vi "Keithley 2002 ACI Config.vi"(0 "GPIB address":string="16", 1 "integration time (0:auto)":u16(ring) items=["automatic", "automatic once", "set to minimum", "set to maximum", "set aperature value", "set NPLC value"], 2 "integ. value":dbl=0.01667 format="%^.2e", 3 "range (auto:0)":u16(ring) items=["autorange", "autorange once", "set min range", "set max range", "set range value"], 4 "range value (amps)":dbl=2.0 min=0.0002 max=2.0 format="%^.2e", 5 "error in":T1, 6 "coupling":bool=TRUE, 7 "resolution (4.5 digits:3)":u16(ring)=3 items=["auto resolution", "auto resolution once", "3.5 digits", "4.5 digits", "5.5 digits", "6.5 digits", "7.5 digits", "8.5 digits"], 8 "reference (off:0)":u16(ring) items=["off", "set reference value"], 9 "digital filter (off:0)":u16(ring) items=["off", "auto filter", "auto filter once", "moving filter", "repeating filter"], 10 "reference value (amps)":dbl min=-2.1 max=2.1 format="%^.2e", 11 "dig. filter count":dbl=10.0 min=1.0 max=100.0 step=1.0 format="%^.2e", 14 "advanced filter (off:0)":u16(ring) items=["off", "enabled"], 15 "noise tolerance (%)":dbl=5.0 min=0.0 max=100.0 step=1.0 format="%^.2e", 16 "detector (rms:0)":u16(ring) items=["RMS", "average"]) -> (19 "error out":T1)   [LabVIEW 2020]
doc: "This VI is used to configure the settings for AC current measurements. The instrument can be in any mode when this VI is run. The settings will go into effect and the instrument will go into the AC current mode."
panel:
  # "ac\ndc"
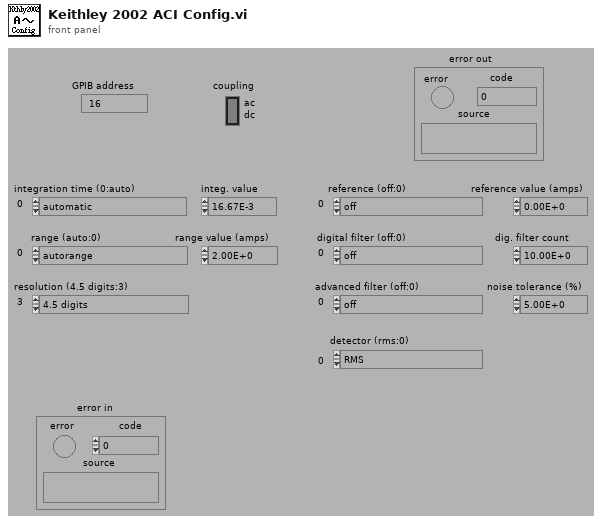
[diagram p1: front panel]
types:
  T1 = cluster{"error":bool, "code":i32, "source":string}
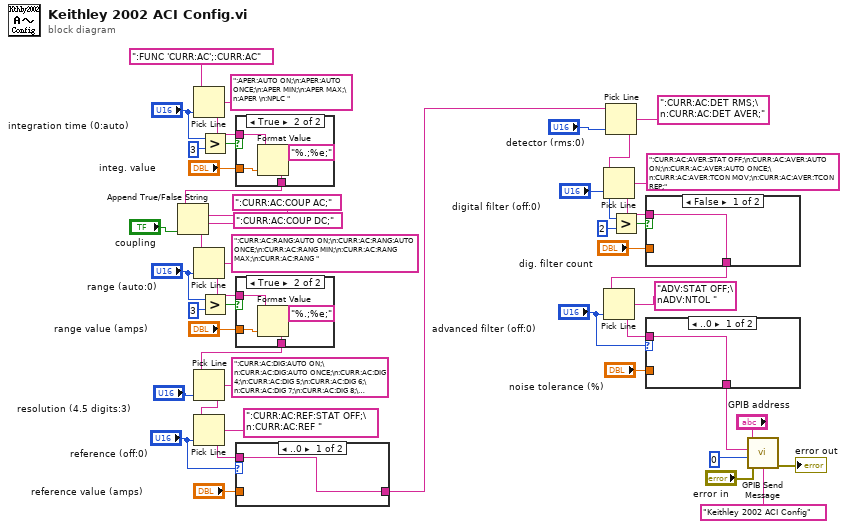
[diagram p0: block diagram]
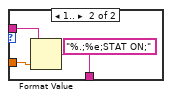
[diagram p2: hidden frame]
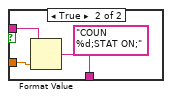
[diagram p3: hidden frame]
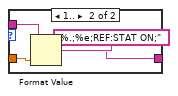
[diagram p4: hidden frame]
diagram:
  n1 = Pick Line(string ("")=":FUNC 'CURR:AC';:CURR:AC", multi-line string=":APER:AUTO ON;\n:APER:AUTO ONCE;\n:APER MIN;\n:APER MAX;\n:APER \n:NPLC ", line index="integration time (0:auto)") -> (output string=w41:string)
  n2 = Greater?(x="integration time (0:auto)", y=3) -> (0:w42:bool)
  n3 = Greater?(x="range (auto:0)", y=3) -> (0:w39:bool)
  n4 = case shown="True" w42 {
    tunnel: "integ. value" -> [_ w51]
    tunnel: w41 -> [w48 w50]
    tunnel: [w48 w49] -> w6
    frame False {
    }
    frame True {
      n5 = Format Value(string ("")=w50, format string="%.;%e;", value (0)=w51) -> (output string=w49:string)
    }
  }
  n6 = Append True/False String(1:"coupling", 2:":CURR:AC:COUP DC;", 3:":CURR:AC:COUP AC;", 4:w6) -> (0:w5:string)
  n7 = Pick Line(string ("")=w5, multi-line string=":CURR:AC:RANG:AUTO ON;\n:CURR:AC:RANG:AUTO ONCE;\n:CURR:AC:RANG MIN;\n:CURR:AC:RANG MAX;\n:CURR:AC:RANG ", line index="range (auto:0)") -> (output string=w40:string)
  n8 = case shown="True" w39 {
    tunnel: "range value (amps)" -> [_ w56]
    tunnel: w40 -> [w53 w55]
    tunnel: [w53 w54] -> w32
    frame False {
    }
    frame True {
      n9 = Format Value(string ("")=w55, format string="%.;%e;", value (0)=w56) -> (output string=w54:string)
    }
  }
  n10 = Pick Line(string ("")=w32, multi-line string=":CURR:AC:DIG:AUTO ON;\n:CURR:AC:DIG:AUTO ONCE;\n:CURR:AC:DIG 4;\n:CURR:AC:DIG 5;\n:CURR:AC:DIG 6;\n:CURR:AC:DIG 7;\n:CURR:AC:DIG 8;\n:Curr:AC:Dig 9;", line index="resolution (4.5 digits:3)") -> (output string=w28:string)
  n11 = Pick Line(string ("")=w28, multi-line string=":CURR:AC:REF:STAT OFF;\n:CURR:AC:REF ", line index="reference (off:0)") -> (output string=w31:string)
  n12 = case shown="..0" "reference (off:0)" {
    tunnel: "reference value (amps)" -> [_ w62]
    tunnel: w31 -> [w58 w61]
    tunnel: [w58 w59] -> w2
    frame ..0 {
    }
    frame 1.. {
      n13 = Format Value(string ("")=w61, format string="%.;%e;REF:STAT ON;", value (0)=w62) -> (output string=w59:string)
    }
  }
  n14 = Pick Line(string ("")=w2, multi-line string=":CURR:AC:DET RMS;\n:CURR:AC:DET AVER;", line index="detector (rms:0)") -> (output string=w1:string)
  n15 = Pick Line(string ("")=w1, multi-line string=":CURR:AC:AVER:STAT OFF;\n:CURR:AC:AVER:AUTO ON;\n:CURR:AC:AVER:AUTO ONCE;\n:CURR:AC:AVER:TCON MOV;\n:CURR:AC:AVER:TCON REP;", line index="digital filter (off:0)") -> (output string=w25:string)
  n16 = Greater?(x="digital filter (off:0)", y=2) -> (0:w22:bool)
  n17 = case shown="False" w22 {
    tunnel: "dig. filter count" -> [_ w67]
    tunnel: w25 -> [w63 w66]
    tunnel: [w63 w65] -> w14
    frame False {
    }
    frame True {
      n18 = Format Value(string ("")=w66, format string="COUN %d;STAT ON;", value (0)=w67) -> (output string=w65:string)
    }
  }
  n19 = Pick Line(string ("")=w14, multi-line string="ADV:STAT OFF;\nADV:NTOL ", line index="advanced filter (off:0)") -> (output string=w18:string)
  n20 = case shown="..0" "advanced filter (off:0)" {
    tunnel: "noise tolerance (%)" -> [_ w72]
    tunnel: w18 -> [w68 w71]
    tunnel: [w68 w70] -> w15
    frame ..0 {
    }
    frame 1.. {
      n21 = Format Value(string ("")=w71, format string="%.;%e;STAT ON;", value (0)=w72) -> (output string=w70:string)
    }
  }
  n22 = call "GPIB Send Message.vi"("address string"="GPIB address", "write buffer"=w15, "source"="Keithley 2002 ACI Config", "write mode (set END:0)"=0, "error in"="error in") -> ("error out"=→"error out":T1)  [unwired: 2 in, 2 out]
